vi "Lookup Service.vi"(7 "Service Lookup":refnum<class "Service.lvclass">, 8 "error in (no error)":errorcluster, 11 "Service Container in":refnum<class "Service Container.lvclass">) -> (0 "error out":errorcluster, 2 "Service":refnum<class "Service.lvclass">, 3 "Service Container out":refnum<class "Service Container.lvclass">)   [LabVIEW 2020, in "Vecto.lvlib" / "Service Container.lvclass"]
uses:
  Service Container.lvclass
  Service/Service.lvclass
  Service Container.lvclass/Service Container.ctl
  <vilib>/Utility/error.llb/Error Cluster From Error Code.vi
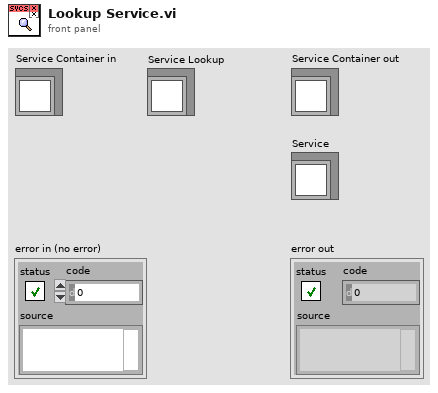
[diagram p1: front panel]
types:
  T1 = typedef "Vecto.lvlib/Service Container.lvclass/Services.ctl" = map{string, map{string, refnum<class "Service.lvclass">}}
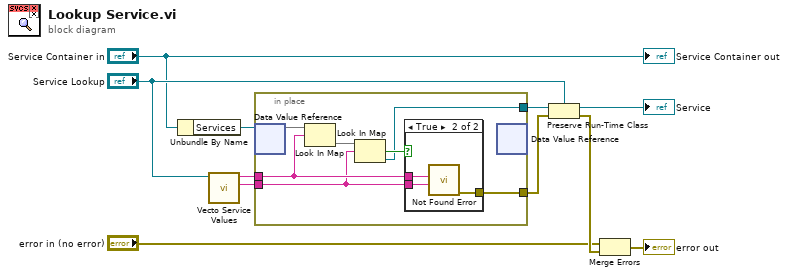
[diagram p0: block diagram]
diagram:
  n1 = Unbundle By Name("Service Container in") -> ("Services"=w11:refnum<data-value>)
  n2 = call "Vecto Service Values.vi"("Service in"="Service Lookup") -> ("ID"=w9:string, "Type"=w10:string)  [unwired: 9 in]
  n3 = in-place {
    in-place-border: w10 -> [w14]
    in-place-border: w9 -> [w13]
    in-place-border: [w15] -> w5
    in-place-border: [w12] -> w4
    n4 = in-place-dvr #1(w11) -> (w18:T1)  [unwired: 1 out]
    n5 = Look In Map(map=w18, key=w14) -> (value=w17:map{string, refnum<class "Service.lvclass">})  [unwired: 1 in, 1 out]
    n6 = Look In Map(map=w17, key=w13) -> (key not found?=w16:bool, value=w15:refnum<class "Service.lvclass">)  [unwired: 1 in]
    n7 = case shown="True" w16 {
      tunnel: w14 -> [_ w21]
      tunnel: w13 -> [_ w20]
      tunnel: [_ w19] -> w12
      frame False {
      }
      frame True {
        n8 = call "Not Found Error.vi"("ID"=w20, "Type"=w21) -> ("error out"=w19:errorcluster)  [unwired: 9 in]
      }
    }
    n9 = in-place-dvr #1() -> ()  [unwired: 1 in, 2 out]
  }
  n10 = Preserve Run-Time Class(object in=w5, error in=w4, 2:"Service Lookup") -> (object out=→"Service":refnum<class "Service.lvclass">, error out=w3:errorcluster)
  n11 = Merge Errors("error in (no error)", w3) -> (→"error out":errorcluster)
  "Service Container out" <- "Service Container in"
